vi "Bypass Lid Redundancy.vi"(0 "GEA2 Reference In":refnum<k24>, 11 "Error In":errorcluster) -> (4 "GEA2 Reference Out":refnum<k24>, 6 "Pass/Fail?":bool=TRUE, 8 "Report Text":string, 15 "Error Out":errorcluster)   [LabVIEW 2016, in "Centauro.lvlib"]
doc: "Use this VI to bypass lid redundancy check by write non 0 to operating mode."
uses:
  Projects/Centauro.lvlib
  Q:/Common/DLLs/GEA3/GeaCommunication.dll
  Common/DLLs/GEA3/GeaCommunication.dll
  Common/LabVIEW GEA2 Toolkit/LabVIEW_GEA2_Toolkit.lvlibp/type defs/Source_Destination.ctl
  Common/LabVIEW GEA2 Toolkit/LabVIEW_GEA2_Toolkit.lvlibp/type defs/ERD Read Data In.ctl
  Common/LabVIEW GEA2 Toolkit/LabVIEW_GEA2_Toolkit.lvlibp/type defs/Data Type.ctl
  Common/LabVIEW GEA2 Toolkit/LabVIEW_GEA2_Toolkit.lvlibp/type defs/ERD Write Data In.ctl
  Common/LabVIEW GEA2 Toolkit/LabVIEW_GEA2_Toolkit.lvlibp
panel:
  in  "Standalone?":bool
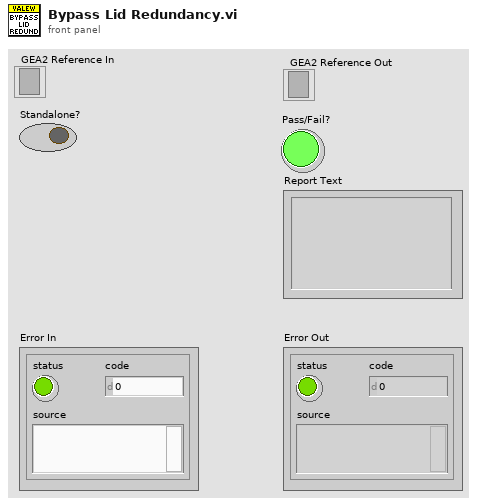
[diagram p1: front panel]
types:
  T1 = typedef "LabVIEW_GEA2_Toolkit.lvlibp/ERD Write Data In.ctl" = cluster{"ERD Number":u16, "Data Type":T2, "Data":string}
  T2 = typedef "LabVIEW_GEA2_Toolkit.lvlibp/Data Type.ctl" = enum16{"string", "boolean", "uint8_t", "uint16_t", "uint32_t", "uint64_t", "int8_t", "int16_t", "int32_t", "int64_t"}
  T3 = typedef "LabVIEW_GEA2_Toolkit.lvlibp/ERD Read Data In.ctl" = cluster{"ERD Number":u16, "Data Type":T2}
  T4 = typedef "LabVIEW_GEA2_Toolkit.lvlibp/Source_Destination.ctl" = cluster{"Source":u8, "Destination":u8}
  T5 = typedef "LabVIEW_GEA2_Toolkit.lvlibp/ERD Read Data Out.ctl" = cluster{"ERD Number":u16, "Data":string}
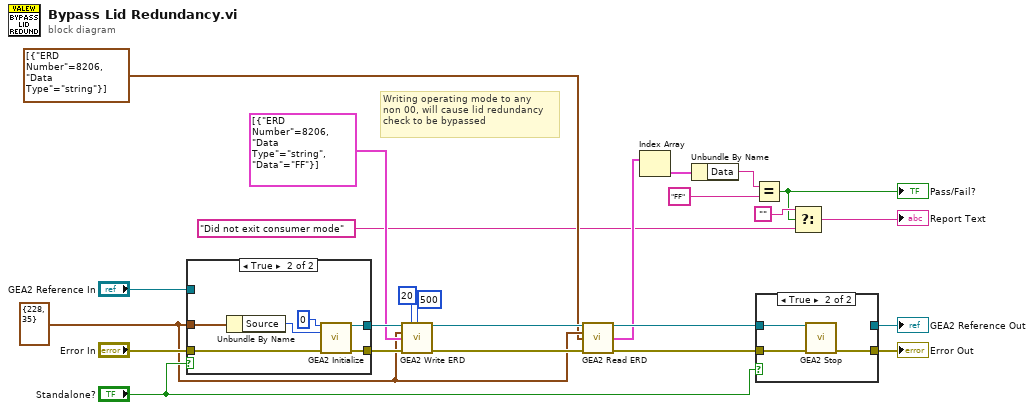
[diagram p0: block diagram]
diagram:
  w14 = T4 {"Source"=228, "Destination"=35} ("GEA Inputs")
  # "Writing operating mode to any\nnon 00, will cause lid redundancy\ncheck to be bypassed"
  n1 = case shown="True" "Standalone?" {
    tunnel: "Error In" -> [w25 w32]
    tunnel: [w25 w31] -> w18
    tunnel: "GEA2 Reference In" -> [w26 _]
    tunnel: [w26 w30] -> w24
    tunnel: w14 -> [_ w28]
    frame False {
    }
    frame True {
      n2 = Unbundle By Name(w28) -> ("Source"=w29:u8)
      n3 = call "GEA2 Initialize.vi"("Board Index"=0, "Source Address"=w29, "error in"=w32) -> ("GEA2 Reference Out"=w30:refnum<k24>, "error out"=w31:errorcluster)  [unwired: 10 in, 1 out]
    }
  }
  n4 = call "GEA2 Write ERD.vi"("GEA2 Reference In"=w24, "# of Tries"=u8 20, "Read Timeout (ms)"=u32 500, "GEA Inputs"=w14, "Write ERD List"=T1[] [{"ERD Number"=8206, "Data Type"=enum."string", "Data"="FF"}], "Error In"=w18) -> ("GEA2 Reference Out"=w16:refnum<k24>, "Error Out"=w15:errorcluster)  [unwired: 7 in, 1 out]
  n5 = call "GEA2 Read ERD.vi"("GEA2 Reference In"=w16, "GEA Inputs"=w14, "Read ERD List"=T3[] [{"ERD Number"=8206, "Data Type"=enum."string"}], "Error In"=w15) -> ("GEA2 Reference Out"=w12:refnum<k24>, "ERD Data Out"=w8:T5[], "Error Out"=w11:errorcluster)  [unwired: 8 in, 1 out]
  n6 = Index Array(array=w8) -> (element=w7:T5)  [unwired: 1 in]
  n7 = Unbundle By Name(w7) -> ("Data"=w6:string)
  n8 = Equal?(x=w6, y="FF") -> (x = y?=w5:bool)
  "Pass/Fail?" <- w5
  n9 = case shown="True" "Standalone?" {
    tunnel: w11 -> [w34 w37]
    tunnel: [w34 w36] -> w23
    tunnel: [w33 _] -> w22
    tunnel: w12 -> [w33 w35]
    frame False {
    }
    frame True {
      n10 = call "GEA2 Stop.vi"("GEA2 Reference In"=w35, "Error In"=w37) -> ("Error Out"=w36:errorcluster)  [unwired: 13 in]
    }
  }
  "Error Out" <- w23
  "GEA2 Reference Out" <- w22
  n11 = Select(t="", s=w5, f="Did not exit consumer mode") -> (s? t:f=→"Report Text":string)
